vi "DIAdem Close Connection.vi"(8 "error in (no error)":errorcluster, 11 "DIAdem Reference":T1) -> (0 "error out":errorcluster)   [LabVIEW 2020]
doc: "This VI closes the reference to the DIAdem application. The DIAdem environment is closed if it was not originally open."
uses:
  <vilib>/ExportToExcel/DIAdem Reference.ctl
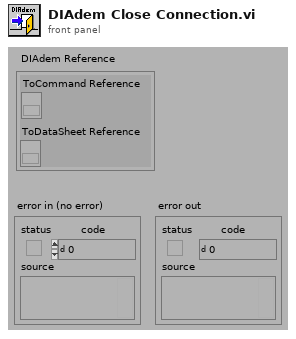
[diagram p1: front panel]
types:
  T1 = typedef "DIAdem Reference.ctl" = cluster{"ToCommand Reference":refnum<k7>, "ToDataSheet Reference":refnum<k7>}
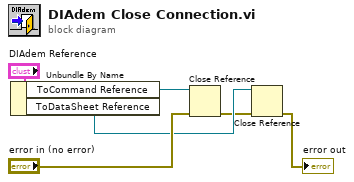
[diagram p0: block diagram]
diagram:
  n1 = Unbundle By Name("DIAdem Reference") -> ("ToCommand Reference"=w4:refnum<k7>, "ToDataSheet Reference"=w3:refnum<k7>)
  n2 = Close Reference(reference=w4, error in (no error)="error in (no error)") -> (error out=w2:errorcluster)
  n3 = Close Reference(reference=w3, error in (no error)=w2) -> (error out=→"error out":errorcluster)
